vi "aggState.vi"(8 "error in (no error)":errorcluster, 9 "dofIdx":i32[](array[numeric]), 10 "State in DOF":dbl[](array[numeric]), 11 "OptCtrl in":refnum<class "OptCtrl.lvclass">) -> (0 "error out":errorcluster, 3 "OptCtrl out":refnum<class "OptCtrl.lvclass">)   [LabVIEW 2016, in "OptCtrl.lvclass"]
doc: "Aggregate the calculate degree of freedom (DOF) in the state."
uses:
  OptCtrl.lvclass
  OptCtrl.lvclass/OptCtrl.ctl
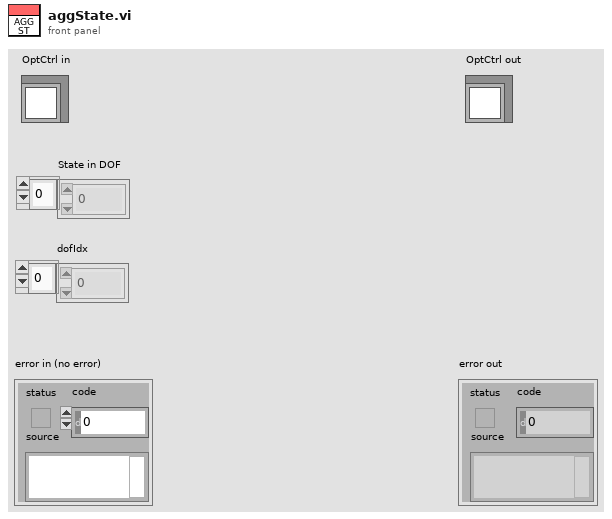
[diagram p1: front panel]
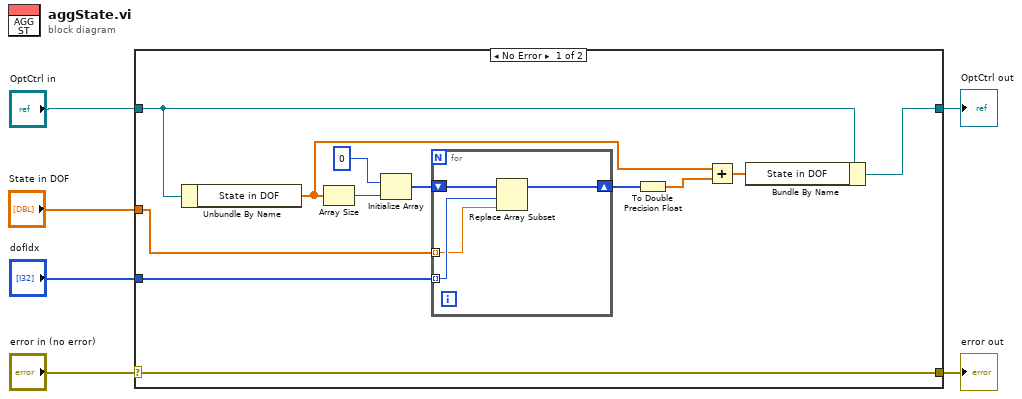
[diagram p0: block diagram]
diagram:
  n1 = case shown="No Error" "error in (no error)" {
    selector: "error in (no error)" -> [w18 w24]
    tunnel: [w18 w24] -> w5
    tunnel: [w7 w23] -> w4
    tunnel: "OptCtrl in" -> [w8 w23]
    tunnel: "dofIdx" -> [w14 _]
    tunnel: "State in DOF" -> [w13 _]
    frame No Error {
      n2 = Unbundle By Name(w8) -> ("State in DOF"=w12:dbl[])
      n3 = Array Size(array=w12) -> (size(s)=w17:i32)
      n4 = Initialize Array(0 ("element"), w17) -> (w15:i32[])
      n5 = for {
        tunnel: w14 -> [w21] mode=indexing
        tunnel: w13 -> [w20] mode=indexing
        shift-right: [w19] -> w11
        shift-left: w15 -> [w22]
        n6 = Replace Array Subset(array=w22, new element=w20, index=w21) -> (w19:i32[])
      }
      n7 = To Double Precision Float(number=w11) -> (double precision float=w10:dbl[])
      n8 = Add(x=w12, y=w10) -> (x+y=w9:dbl[])
      n9 = Bundle By Name(cluster=w8, "State in DOF"=w9) -> (w7:refnum<class "OptCtrl.lvclass">)
    }
    frame Error {
    }
  }
  "error out" <- w5
  "OptCtrl out" <- w4
